vi "_SearchPeakList.vi"(5 "Search Window (3)":dbl=3.0 min=0.1 format="%#.6f", 6 "Peak List":T1[](array[typedef]), 7 "RefMass":dbl) -> (0 "Valid Peak?":bool, 1 "Found 2":bool, 2 "Peak":T1, 3 "Found":bool)   [LabVIEW 2015]
uses:
  Type/_Peak Property.ctl
panel:
  # "(after searching an expanded window)"
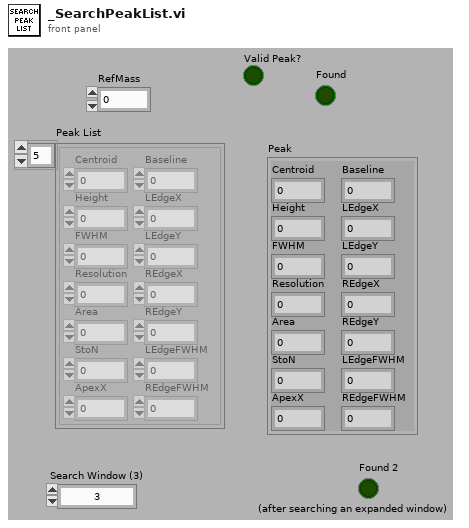
[diagram p1: front panel]
types:
  T1 = typedef "_Peak Property.ctl" = cluster{"Centroid":dbl, "Height":dbl, "FWHM":dbl, "Resolution":dbl, "Area":dbl, "StoN":dbl, "ApexX":dbl, "Baseline":dbl, "LEdgeX":dbl, "LEdgeY":dbl, "REdgeX":dbl, "REdgeY":dbl, "LEdgeFWHM":dbl, "REdgeFWHM":dbl}
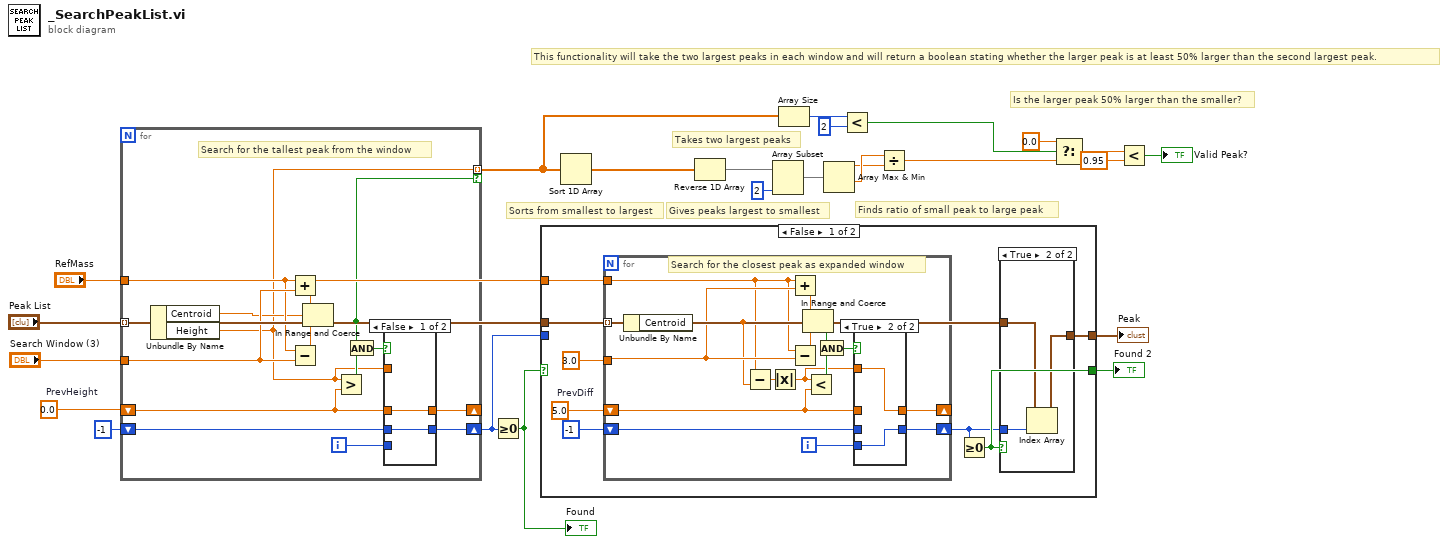
[diagram p0: block diagram]
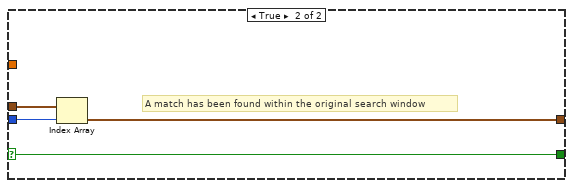
[diagram p4: hidden frame]
diagram:
  w22 = 0.0  # PrevHeight
  # "Is the larger peak 50% larger than the smaller?"
  # "Takes two largest peaks"
  # "Finds ratio of small peak to large peak"
  # "Gives peaks largest to smallest"
  # "Sorts from smallest to largest"
  # "This functionality will take the two largest peaks in each window and will return a boolean stating whether the larger peak is at least 50% larger than the second largest peak."
  n1 = for {
    tunnel: "Peak List" -> [w39] mode=indexing
    tunnel: "RefMass" -> [w35]
    shift-right: [w30] -> _
    shift-left: w22 -> [w31]
    tunnel: "Search Window (3)" -> [w36]
    shift-right: [w28] -> w18
    shift-left: -1 -> [w29]
    tunnel: [w26] -> w2 mode=indexing if=w25
    i -> [w27]
    # "Search for the tallest peak from the window"
    n2 = Unbundle By Name(w39) -> ("Centroid"=w34:dbl, "Height"=w26:dbl)
    n3 = Add(x=w35, y=w36) -> (x+y=w37:dbl)
    n4 = Subtract(x=w35, y=w36) -> (x-y=w38:dbl)
    n5 = In Range and Coerce(upper limit=w37, x=w34, lower limit=w38) -> (In Range?=w25:bool)  [unwired: 1 out]
    n6 = Greater?(x=w26, y=w31) -> (0:w33:bool)
    n7 = And(x=w25, y=w33) -> (x .and. y?=w32:bool)
    n8 = case shown="False" w32 {
      tunnel: [w41 w42] -> w30
      tunnel: w31 -> [w41 _]
      tunnel: [w40 w43] -> w28
      tunnel: w29 -> [w40 _]
      tunnel: w26 -> [_ w42]
      tunnel: w27 -> [_ w43]
      frame False {
      }
      frame True {
      }
    }
  }
  n9 = Greater Or Equal To 0?(x=w18) -> (x >= 0?=w21:bool)
  "Found" <- w21
  n10 = case shown="False" w21 {
    selector: w21 -> [_ w78]
    tunnel: [w44 w75] -> w20
    tunnel: [w47 w78] -> w19
    tunnel: "Peak List" -> [w45 w77]
    tunnel: w18 -> [_ w76]
    tunnel: "RefMass" -> [w51 _]
    frame False {
      w48 = 5.0  # PrevDiff
      n11 = for {
        tunnel: w45 -> [w70] mode=indexing
        tunnel: w51 -> [w58]
        shift-right: [w62] -> _
        shift-left: w48 -> [w63]
        tunnel: 3.0 ("Search Window (3)") -> [w67]
        shift-right: [w60] -> w46
        shift-left: -1 -> [w61]
        i -> [w59]
        # "Search for the closest peak as expanded window"
        n12 = Unbundle By Name(w70) -> ("Centroid"=w57:dbl)
        n13 = Subtract(x=w58, y=w57) -> (x-y=w55:dbl)
        n14 = Absolute Value(x=w55) -> (abs(x)=w56:dbl)
        n15 = Add(x=w58, y=w67) -> (x+y=w68:dbl)
        n16 = Subtract(x=w58, y=w67) -> (x-y=w69:dbl)
        n17 = In Range and Coerce(upper limit=w68, x=w57, lower limit=w69) -> (In Range?=w66:bool)  [unwired: 1 out]
        n18 = Less?(x=w56, y=w63) -> (x < y?=w65:bool)
        n19 = And(x=w66, y=w65) -> (x .and. y?=w64:bool)
        n20 = case shown="True" w64 {
          tunnel: [w72 w73] -> w62
          tunnel: w63 -> [w72 _]
          tunnel: [w71 w74] -> w60
          tunnel: w61 -> [w71 _]
          tunnel: w56 -> [_ w73]
          tunnel: w59 -> [_ w74]
          frame False {
          }
          frame True {
          }
        }
      }
      n21 = Greater Or Equal To 0?(x=w46) -> (x >= 0?=w47:bool)
      n22 = case shown="True" w47 {
        tunnel: w46 -> [_ w54]
        tunnel: w45 -> [_ w53]
        tunnel: [_ w52] -> w44
        frame False {
        }
        frame True {
          n23 = Index Array(array=w53, index=w54) -> (element=w52:T1)
        }
      }
    }
    frame True {
      # "A match has been found within the original search window"
      n24 = Index Array(array=w77, index=w76) -> (element=w75:T1)
    }
  }
  "Found 2" <- w19
  "Peak" <- w20
  n25 = Sort 1D Array(array=w2) -> (sorted array=w15:dbl[])
  n26 = Reverse 1D Array(array=w15) -> (reversed array=w13:dbl[])
  n27 = Array Subset(array=w13, length=2) -> (w12:dbl[])  [unwired: 1 in]
  n28 = Array Size(array=w2) -> (size(s)=w8:i32)
  n29 = Array Max & Min(array=w12) -> (max value=w10:dbl, min value=w11:dbl)  [unwired: 2 out]
  n30 = Less?(x=w8, y=2) -> (x < y?=w6:bool)
  n31 = Divide(x=w11, y=w10) -> (x/y=w9:dbl)
  n32 = Select(t=0.0, s=w6, f=w9) -> (s? t:f=w4:dbl)
  n33 = Less?(x=w4, y=0.95) -> (x < y?=→"Valid Peak?":bool)
